vi "Tree_FocusArrayPath_Tests.vi"(11 "error in":errorcluster) -> (15 "error out":errorcluster)   [LabVIEW 2016, in "DronaTest.lvlib"]
uses:
  DronaTest.lvlib
  APIs/Stimulus/ControlValue/SetValueAuto.vi
  APIs/Stimulus/ControlValue/Controls/Tree/SetValueByHierarchicalPathArray.vi
  APIs/Assert/AssertControlValue/Controls/Tree/AssertValueByArrayPath.vi
  <vilib>/addons/_JKI Toolkits/Caraya/classes/Assert/Assert Error.vi
  <vilib>/addons/_JKI Toolkits/Caraya/classes/Assert/Assert Equal Value_Variant.vi
  <vilib>/addons/_JKI Toolkits/Caraya/classes/Test/Test.lvclass
  Drona.lvlib
  <vilib>/SLL Toolkit/SLL Debug/SLL Debug.lvlib
  APIs/Stimulus/ControlValue/ControlValue.lvlib
  <vilib>/addons/_JKI Toolkits/Caraya/classes/Assert/Assert.lvclass
  APIs/Stimulus/ControlValue/Controls/Tree/StimulusTree.lvlib
  APIs/Assert/AssertControlValue/Controls/Tree/AssertTree.lvlib
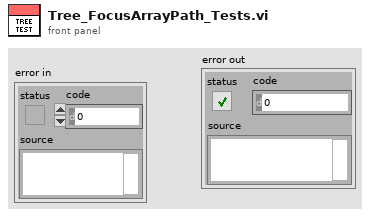
[diagram p1: front panel]
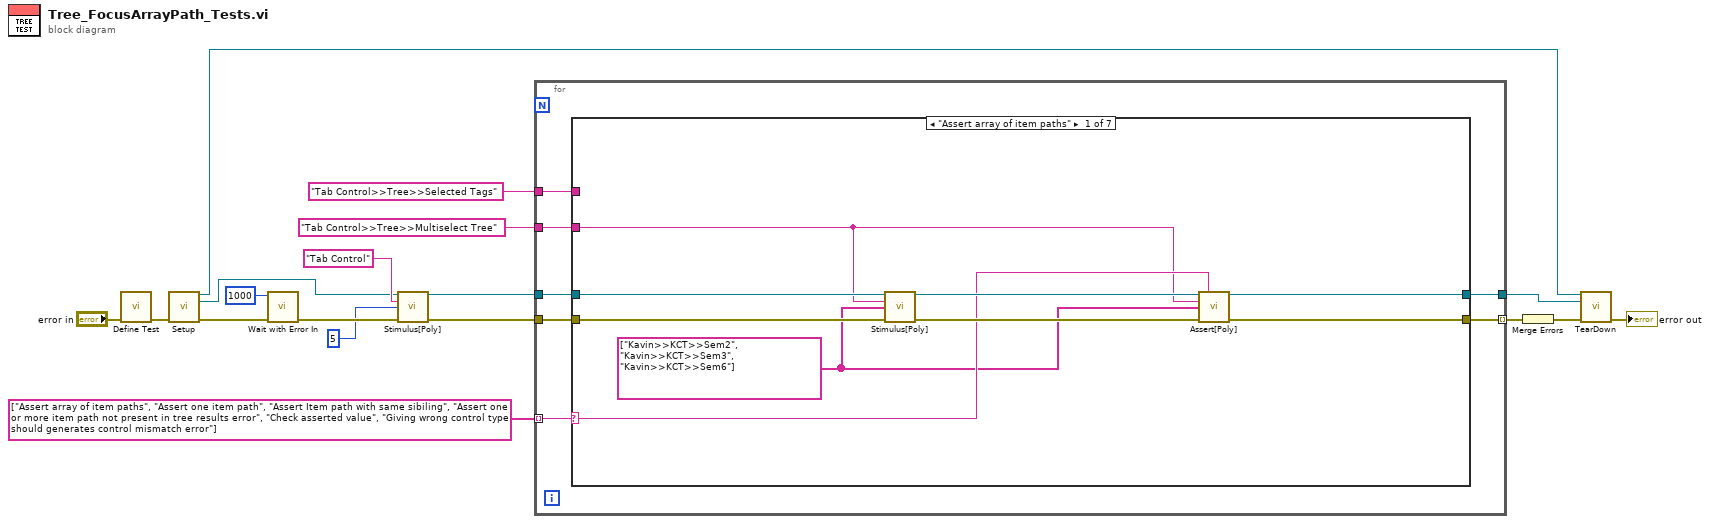
[diagram p0: block diagram]
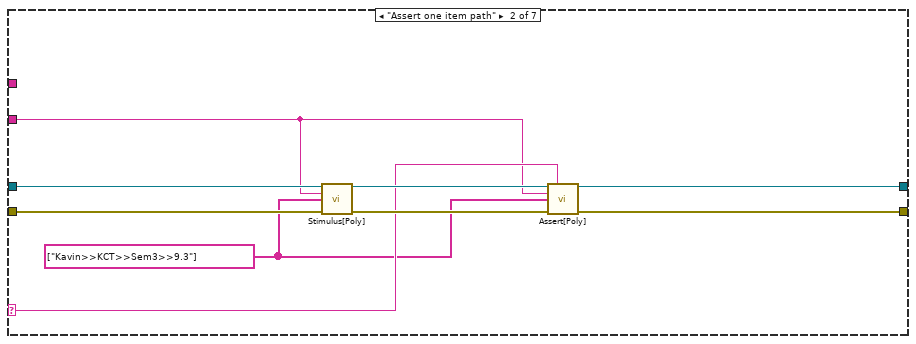
[diagram p2: hidden frame]
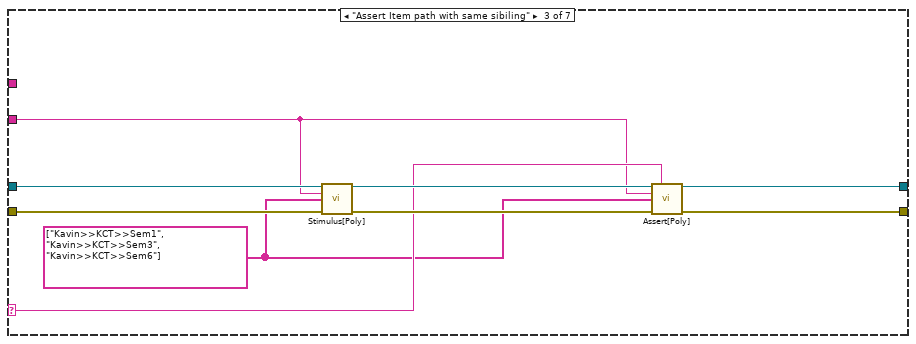
[diagram p3: hidden frame]
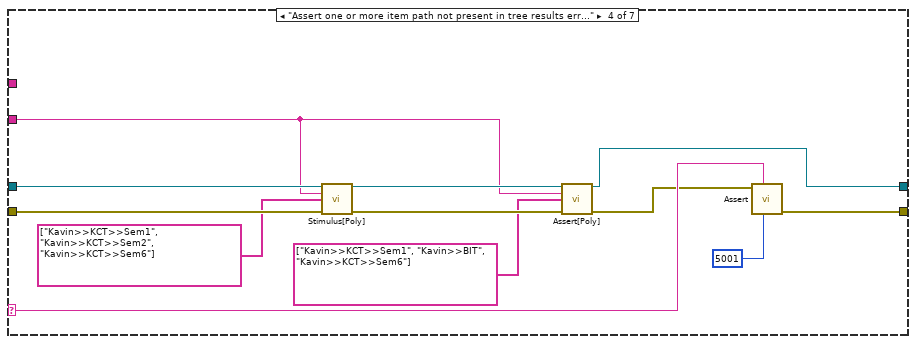
[diagram p4: hidden frame]
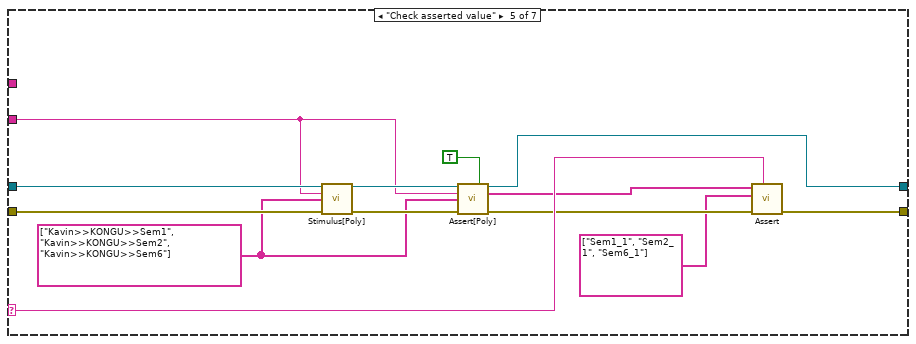
[diagram p5: hidden frame]
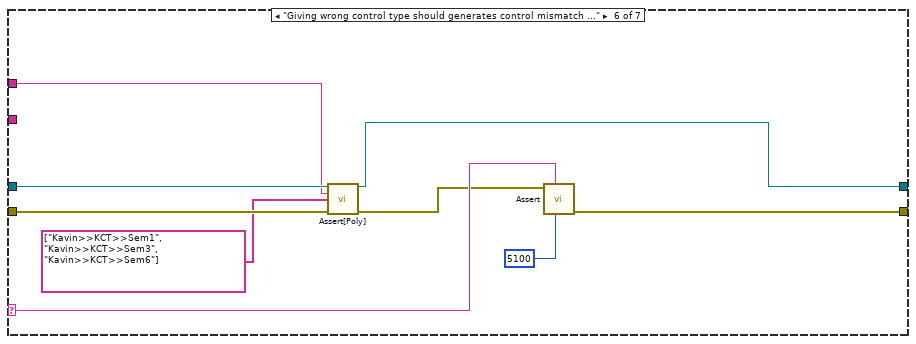
[diagram p6: hidden frame]
diagram:
  n1 = call <vilib>:"Define Test.vi"("error in (no error)"="error in") -> ("error out"=w7:errorcluster)  [unwired: 10 in]
  n2 = call "Setup.vi"("error in (no error)"=w7) -> ("Application Ref"=w2:refnum<vi>, "VI out"=w6:refnum<vi>, "error out"=w5:errorcluster)  [unwired: 12 in]
  n3 = call <vilib>:"Wait with Error In.vi"("error in (no error)"=w5, "milliseconds to wait"=u32 1000) -> ("error out"=w16:errorcluster)  [unwired: 9 in]
  n4 = call-poly "Stimulus[Poly].vi"("VI Reference In"=w6, "Control Path"="Tab Control", "Value (Signaling)"=5, "error in"=w16) -> ("VI Reference Out"=w12:refnum<vi>, "error out"=w15:errorcluster)  [unwired: 10 in]
  n5 = for {
    tunnel: w12 -> [w24]
    tunnel: "Tab Control>>Tree>>Multiselect Tree" ("Control Path") -> [w23]
    tunnel: "Tab Control>>Tree>>Selected Tags" ("Control Path") -> [w22]
    tunnel: string[] ["Assert array of item paths", "Assert one item path", "Assert Item path with same sibiling", "Assert one or more item path not present in tree results error", "Check asserted value", "Giving wrong control type should generates control mismatch error"] -> [w20] mode=indexing
    tunnel: [w19] -> w3
    tunnel: w15 -> [w25]
    tunnel: [w21] -> w8 mode=indexing
    n6 = case shown="\"Assert array of item paths\"" w20 {
      selector: w20 -> [w28 w37 w46 w61 w74 w85 _]
      tunnel: w25 -> [w34 w43 w52 w64 w77 w83 w88]
      tunnel: w24 -> [w33 w42 w51 w63 w76 w81 w87]
      tunnel: w23 -> [w27 w36 w45 w55 w71 _ _]
      tunnel: w22 -> [_ _ _ _ _ w80 _]
      tunnel: [w30 w39 w48 w62 w75 w86 w88] -> w21
      tunnel: [w29 w38 w47 w54 w70 w78 w87] -> w19
      frame "Assert array of item paths" {
        w26 = string[] ["Kavin>>KCT>>Sem2", "Kavin>>KCT>>Sem3", "Kavin>>KCT>>Sem6"] ("Hierarchical Path Array")
        n7 = call-poly "Stimulus[Poly].vi"("VI Reference In"=w33, "Control Path"=w27, "Hierarchical Path Array"=w26, "Error In"=w34) -> ("VI Reference Out"=w31:refnum<vi>, "Error Out"=w32:errorcluster)  [unwired: 10 in]
        n8 = call-poly "Assert[Poly].vi"("VI Reference In"=w31, "Test Label"=w28, "Control Path"=w27, "Focus Item Path"=w26, "Error In"=w32) -> ("VI Reference Out"=w29:refnum<vi>, "Error Out"=w30:errorcluster)  [unwired: 8 in, 1 out]
      }
      frame "Assert one item path" {
        w35 = string[] ["Kavin>>KCT>>Sem3>>9.3"] ("Item Name")
        n9 = call-poly "Stimulus[Poly].vi"("VI Reference In"=w42, "Control Path"=w36, "Hierarchical Path Array"=w35, "Error In"=w43) -> ("VI Reference Out"=w40:refnum<vi>, "Error Out"=w41:errorcluster)  [unwired: 10 in]
        n10 = call-poly "Assert[Poly].vi"("VI Reference In"=w40, "Test Label"=w37, "Control Path"=w36, "Focus Item Path"=w35, "Error In"=w41) -> ("VI Reference Out"=w38:refnum<vi>, "Error Out"=w39:errorcluster)  [unwired: 8 in, 1 out]
      }
      frame "Assert Item path with same sibiling" {
        w44 = string[] ["Kavin>>KCT>>Sem1", "Kavin>>KCT>>Sem3", "Kavin>>KCT>>Sem6"] ("Hierarchical Path Array")
        n11 = call-poly "Stimulus[Poly].vi"("VI Reference In"=w51, "Control Path"=w45, "Hierarchical Path Array"=w44, "Error In"=w52) -> ("VI Reference Out"=w49:refnum<vi>, "Error Out"=w50:errorcluster)  [unwired: 10 in]
        n12 = call-poly "Assert[Poly].vi"("VI Reference In"=w49, "Test Label"=w46, "Control Path"=w45, "Focus Item Path"=w44, "Error In"=w50) -> ("VI Reference Out"=w47:refnum<vi>, "Error Out"=w48:errorcluster)  [unwired: 8 in, 1 out]
      }
      frame "Assert one or more item path not present in tree results error" {
        n13 = call-poly "Stimulus[Poly].vi"("VI Reference In"=w63, "Control Path"=w55, "Hierarchical Path Array"=string[] ["Kavin>>KCT>>Sem1", "Kavin>>KCT>>Sem2", "Kavin>>KCT>>Sem6"], "Error In"=w64) -> ("VI Reference Out"=w56:refnum<vi>, "Error Out"=w58:errorcluster)  [unwired: 10 in]
        n14 = call-poly "Assert[Poly].vi"("VI Reference In"=w56, "Control Path"=w55, "Focus Item Path"=string[] ["Kavin>>KCT>>Sem1", "Kavin>>BIT", "Kavin>>KCT>>Sem6"] ("Hierarchical Path Array"), "Error In"=w58) -> ("VI Reference Out"=w54:refnum<vi>, "Error Out"=w57:errorcluster)  [unwired: 9 in, 1 out]
        n15 = call-poly <vilib>:"Assert.vi"("error code (1)"=5001, "Label"=w61, "Error?"=w57) -> ("error out"=w62:errorcluster)  [unwired: 8 in]
      }
      frame "Check asserted value" {
        w69 = string[] ["Kavin>>KONGU>>Sem1", "Kavin>>KONGU>>Sem2", "Kavin>>KONGU>>Sem6"] ("Hierarchical Path Array")
        n16 = call-poly "Stimulus[Poly].vi"("VI Reference In"=w76, "Control Path"=w71, "Hierarchical Path Array"=w69, "Error In"=w77) -> ("VI Reference Out"=w72:refnum<vi>, "Error Out"=w73:errorcluster)  [unwired: 10 in]
        n17 = call-poly "Assert[Poly].vi"("VI Reference In"=w72, "Assert Only? (F)"=TRUE, "Control Path"=w71, "Focus Item Path"=w69, "Error In"=w73) -> ("VI Reference Out"=w70:refnum<vi>, "Asserted Value"=w66:string[], "Error Out"=w67:errorcluster)  [unwired: 8 in]
        n18 = call-poly <vilib>:"Assert.vi"("Label"=w74, "error in (no error)"=w67, "Y"=string[] ["Sem1_1", "Sem2_1", "Sem6_1"], "X"=w66) -> ("error out"=w75:errorcluster)  [unwired: 7 in]
      }
      frame "Giving wrong control type should generates control mismatch error" {
        n19 = call-poly "Assert[Poly].vi"("VI Reference In"=w81, "Control Path"=w80, "Focus Item Path"=string[] ["Kavin>>KCT>>Sem1", "Kavin>>KCT>>Sem3", "Kavin>>KCT>>Sem6"] ("Hierarchical Path Array"), "Error In"=w83) -> ("VI Reference Out"=w78:refnum<vi>, "Error Out"=w82:errorcluster)  [unwired: 9 in, 1 out]
        n20 = call-poly <vilib>:"Assert.vi"("error code (1)"=5100, "Label"=w85, "Error?"=w82) -> ("error out"=w86:errorcluster)  [unwired: 8 in]
      }
      frame Default {
      }
    }
  }
  n21 = Merge Errors(w8) -> (w4:errorcluster)
  n22 = call "TearDown.vi"("Application Ref"=w2, "VI in"=w3, "error in (no error)"=w4) -> ("error out"=→"error out":errorcluster)  [unwired: 12 in]
